vi "chartsheet set first sheet.vi"(8 "error in (no error)":errorcluster, 11 "chartsheet":u32) -> (0 "error out":errorcluster)   [LabVIEW 8.6]
doc: "void chartsheet_set_first_sheet(lxw_chartsheet chartsheet);"
uses:
  pending_lvxlsxwriter/xlsxwriter.dll
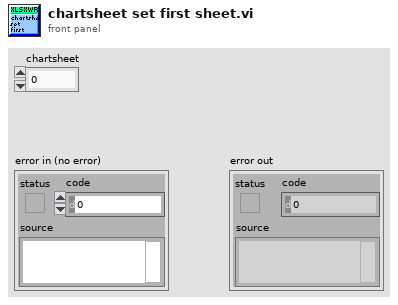
[diagram p1: front panel]
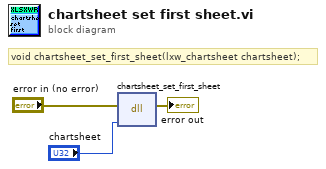
[diagram p0: block diagram]
diagram:
  # "void chartsheet_set_first_sheet(lxw_chartsheet chartsheet);"
  n1 = dll-call lib="C:/Users/WDAGUtilityAccount/Desktop/pending_lvxlsxwriter/xlsxwriter.*" fn="chartsheet_set_first_sheet"(error in="error in (no error)", "chartsheet"="chartsheet") -> (error out=→"error out":errorcluster)  [unwired: 4 in, 1 out]
